vi "Get Caller Coordinates.vi"(0 "Control in":refnum<vi>, 5 "Pane":refnum<vi>, 7 "VI":refnum<vi>, 11 "error in (no error)":errorcluster) -> (4 "Control out":refnum<vi>, 6 "Control Position":T1, 8 "Control Bounds":T2, 15 "error out":errorcluster)   [LabVIEW 2016, in "Code String.lvclass"]
doc: "Calculates the <b>Control Position</b> and <b>Control Bounds</b> in screen coordinates for the <b>Control</b> in <b>Pane</b>.\n--------------------\nCopyright (c) 2019 Analog Devices, Inc. All rights reserved.\n\nRedistribution and use in source and binary forms, with or without modification,\nare permitted provided that the following conditions are met:\n - Redistributions of source code must retain the above copyright notice, this\n list of conditions and the following disclaimer.\n - Redistributions in binary form must reproduce the above copyright notice,\n this list of conditions and the following disclaimer in the documentation\n and/or other materials provided with the distribution.\n - Modified versions of the software must be conspicuously marked as such.\n - This software is licensed solely and exclusively for use with\n processors/products manufactured by or for Analog Devices, Inc.\n - This software may not be combined or merged with other code in any manner\n that would cause the software to become subject to terms and conditions\n which differ from those listed here.\n - Neither the name of Analog Devices, Inc. nor the names of its contributors\n may be used to endorse or promote products derived from this software\n without specific prior written permission.\n - The use of this software may or may not infringe the patent rights of one or\n more patent holders. This license does not release you from the requirement\n that you obtain separate licenses from these patent holders to use this\n software.\n\nTHIS SOFTWARE IS PROVIDED BY ANALOG DEVICES, INC. AND CONTRIBUTORS \"AS IS\" AND\nANY EXPRESS OR IMPLIED WARRANTIES, INCLUDING, BUT NOT LIMITED TO,\nNON-INFRINGEMENT, TITLE, MERCHANTABILITY AND FITNESS FOR A PARTICULAR PURPOSE\nARE DISCLAIMED. IN NO EVENT SHALL ANALOG DEVICES, INC. OR CONTRIBUTORS BE LIABLE\nFOR ANY DIRECT, INDIRECT, INCIDENTAL, SPECIAL, EXEMPLARY, PUNITIVE OR\nCONSEQUENTIAL DAMAGES (INCLUDING, BUT NOT LIMITED TO, DAMAGES ARISING OUT OF\nCLAIMS OF INTELLECTUAL PROPERTY RIGHTS INFRINGEMENT; PROCUREMENT OF SUBSTITUTE\nGOODS OR SERVICES; LOSS OF USE, DATA, OR PROFITS; OR BUSINESS INTERRUPTION)\nHOWEVER CAUSED AND ON ANY THEORY OF LIABILITY, WHETHER IN CONTRACT, STRICT\nLIABILITY, OR TORT (INCLUDING NEGLIGENCE OR OTHERWISE) ARISING IN ANY WAY OUT OF\nTHE USE OF THIS SOFTWARE, EVEN IF ADVISED OF THE POSSIBILITY OF SUCH DAMAGE.\n\n2019-01-10-7CBSD SLA"
uses:
  Code String.lvclass
  <vilib>/Utility/miscctls.llb/LVRectTypeDef.ctl
  <vilib>/Utility/miscctls.llb/LVPointTypeDef.ctl
panel:
  # "Copyright (c) 2019 Analog Devices, Inc.  All rights reserved.\n\nRedistribution and use in source and binary forms, with or without modification,\nare permitted provided that the following conditions are met:\n  - Redistributions of source code must retain the above copyright notice, this\n    list of conditions and the following disclaimer.\n  - Redistributions in binary form must reproduce the above copyright notice,\n    this list of conditions and the following disclaimer in the documentation\n    and/or other materials provided with the distribution.\n  - Modified versions of the software must be conspicuously marked as such.\n  - This software is licensed solely and exclusively for use with\n    processors/products manufactured by or for Analog Devices, Inc.\n  - This software may not be combined or merged with other code in any manner\n    that would cause the software to become subject to terms and conditions\n    which differ from those listed here.\n  - Neither the name of Analog Devices, Inc. nor the names of its contributors\n    may be used to endorse or promote products derived from this software\n    without specific prior written permission.\n  - The use of this software may or may not infringe the patent rights of one or\n    more patent holders.  This license does not release you from the requirement\n    that you obtain separate licenses from these patent holders to use this\n    software.\n\nTHIS SOFTWARE IS PROVIDED BY ANALOG DEVICES, INC. AND CONTRIBUTORS \"AS IS\" AND\nANY EXPRESS OR IMPLIED WARRANTIES, INCLUDING, BUT NOT LIMITED TO,\nNON-INFRINGEMENT, TITLE, MERCHANTABILITY AND FITNESS FOR A PARTICULAR PURPOSE\nARE DISCLAIMED. IN NO EVENT SHALL ANALOG DEVICES, INC. OR CONTRIBUTORS BE LIABLE\nFOR ANY DIRECT, INDIRECT, INCIDENTAL, SPECIAL, EXEMPLARY, PUNITIVE OR\nCONSEQUENTIAL DAMAGES (INCLUDING, BUT NOT LIMITED TO, DAMAGES ARISING OUT OF\nCLAIMS OF INTELLECTUAL PROPERTY RIGHTS INFRINGEMENT; PROCUREMENT OF SUBSTITUTE\nGOODS OR SERVICES; LOSS OF USE, DATA, OR PROFITS; OR BUSINESS INTERRUPTION)\nHOWEVER CAUSED AND ON ANY THEORY OF LIABILITY, WHETHER IN CONTRACT, STRICT\nLIABILITY, OR TORT (INCLUDING NEGLIGENCE OR OTHERWISE) ARISING IN ANY WAY OUT OF\nTHE USE OF THIS SOFTWARE, EVEN IF ADVISED OF THE POSSIBILITY OF SUCH DAMAGE.\n\n2019-01-10-7CBSD SLA"
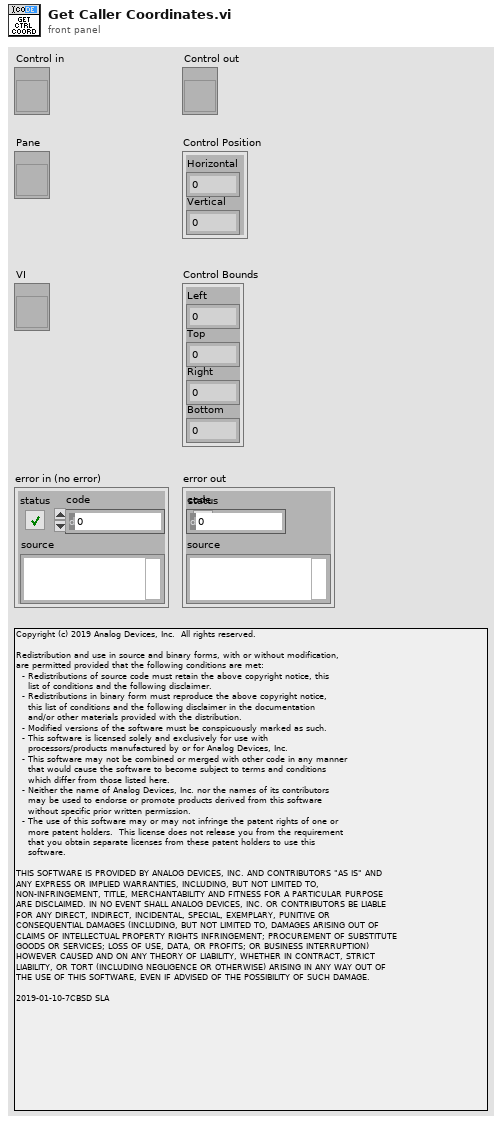
[diagram p1: front panel]
types:
  T1 = typedef "LVPointTypeDef.ctl" = cluster{"Horizontal":i16, "Vertical":i16}
  T2 = typedef "LVRectTypeDef.ctl" = cluster{"Left":i16, "Top":i16, "Right":i16, "Bottom":i16}
  T3 = typedef "LVPositionTypeDef.ctl" = cluster{"Left":i32, "Top":i32}
  T4 = typedef "LVBoundsTypeDef.ctl" = cluster{"Width":u32, "Height":u32}
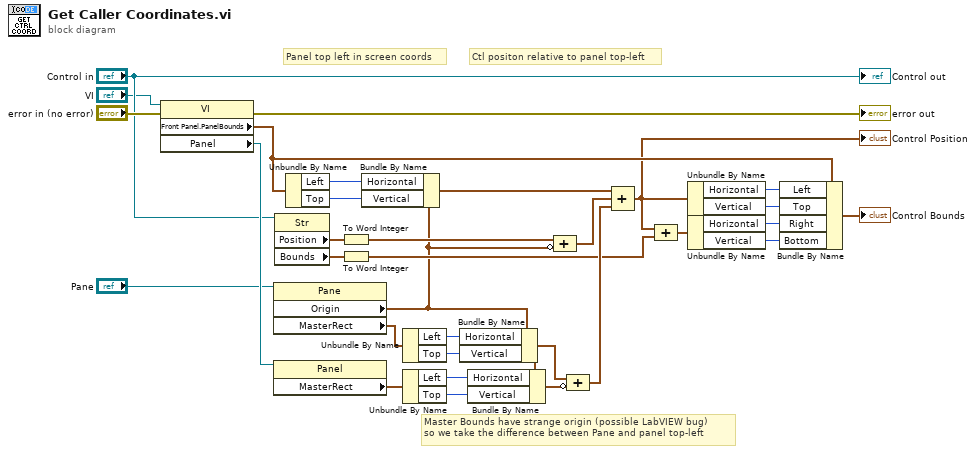
[diagram p0: block diagram]
diagram:
  # "Panel top left in screen coords"
  # "Ctl positon relative to panel top-left"
  # "Master Bounds have strange origin (possible LabVIEW bug)\nso we take the difference between Pane and panel top-left"
  n1 = property on="Property Node" class="VI"(reference="VI", error in="error in (no error)") -> (error out=→"error out":errorcluster, "Front Panel.PanelBounds"=w8:T2, "Panel"=w7:refnum<vi>)  [unwired: 1 out]
  n2 = property on="Property Node" class="Pane"(reference="Pane") -> ("Origin"=w6:T1, "MasterRect"=w23:T2)  [unwired: 1 in, 2 out]
  n3 = property on="Property Node" class="Panel"(reference=w7) -> ("MasterRect"=w15:T2)  [unwired: 1 in, 2 out]
  n4 = property on="Property Node" class="Str"(reference="Control in") -> ("Position"=w31:T3, "Bounds"=w30:T4)  [unwired: 1 in, 2 out]
  n5 = Unbundle By Name(w8) -> ("Left"=w22:i16, "Top"=w21:i16)
  n6 = To Word Integer(number=w31) -> (16bit integer=w10:cluster{"Left":i16, "Top":i16})
  n7 = To Word Integer(number=w30) -> (16bit integer=w9:cluster{"Width":i16, "Height":i16})
  n8 = Bundle By Name(cluster=w6, "Horizontal"=w22, "Vertical"=w21) -> (w18:T1)
  n9 = Unbundle By Name(w23) -> ("Left"=w20:i16, "Top"=w19:i16)
  n10 = Unbundle By Name(w15) -> ("Left"=w16:i16, "Top"=w17:i16)
  n11 = Bundle By Name(cluster=w6, "Horizontal"=w20, "Vertical"=w19) -> (w12:T1)
  n12 = Bundle By Name(cluster=w12, "Horizontal"=w16, "Vertical"=w17) -> (w13:T1)
  n13 = Compound Arithmetic op=ADD(w10, invert w6) -> (w11:T1)
  n14 = Compound Arithmetic op=ADD(w12, invert w13) -> (w14:T1)
  n15 = Compound Arithmetic op=ADD(w18, w11, w14) -> (w4:T1)
  "Control Position" <- w4
  n16 = Compound Arithmetic op=ADD(w4, w9) -> (w25:T1)
  n17 = Unbundle By Name(w4) -> ("Horizontal"=w29:i16, "Vertical"=w28:i16)
  n18 = Unbundle By Name(w25) -> ("Horizontal"=w27:i16, "Vertical"=w26:i16)
  n19 = Bundle By Name(cluster=w8, "Left"=w29, "Top"=w28, "Right"=w27, "Bottom"=w26) -> (→"Control Bounds":T2)
  "Control out" <- "Control in"
